vi "N-Insert.vi"(8 "error in":errorcluster, 10 "Waveform":waveform(dbl)[](array[waveform]), 11 "Q Name":string) -> (0 "error out":errorcluster)   [LabVIEW 2016]
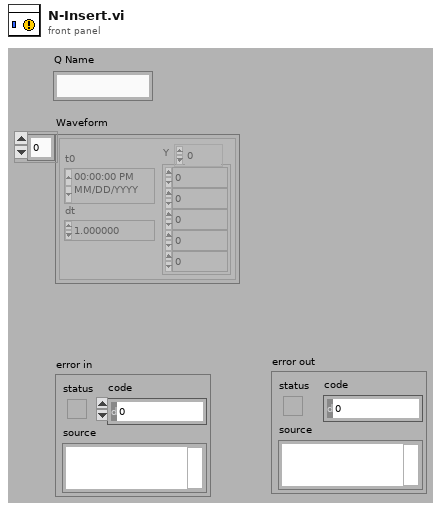
[diagram p1: front panel]
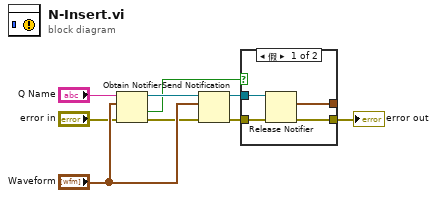
[diagram p0: block diagram]
diagram:
  n1 = Obtain Notifier(name (unnamed)="Q Name", notification data type="Waveform", error in (no error)="error in") -> (notifier out=w8:refnum<notifier>, created new?=w6:bool, error out=w1:errorcluster)  [unwired: 1 in]
  n2 = Send Notification(notification="Waveform", notifier=w8, error in (no error)=w1) -> (notifier out=w5:refnum<notifier>, error out=w4:errorcluster)
  n3 = case shown="假" w6 {
    tunnel: w5 -> [w13 _]
    tunnel: w4 -> [w12 w14]
    tunnel: [w11 w14] -> w3
    tunnel: [w10 _] -> _
    frame False {
      n4 = Release Notifier(notifier=w13, error in (no error)=w12) -> (last notification=w10:waveform(dbl)[], error out=w11:errorcluster)  [unwired: 1 in, 1 out]
    }
    frame True {
    }
  }
  "error out" <- w3
